vi "Test_URI_Class_SetQuery.vi"(8 "error in (no error)":errorcluster) -> (0 "error out":errorcluster)   [LabVIEW 2013]
uses:
  source/utilities/isHEXDigit.vi
  <vilib>/addons/_JKI Toolkits/Caraya/classes/Assert/Assert Equal Value_Variant.vi
  <vilib>/addons/_JKI Toolkits/Caraya/classes/Assert/Assert True.vi
  source/utilities/Extract URI Components.vi
  <vilib>/Utility/error.llb/Trim Whitespace.vi
  <vilib>/addons/_JKI Toolkits/Caraya/classes/Test/Test.lvclass
  <vilib>/addons/_JKI Toolkits/Caraya/classes/Assert/Assert.lvclass
  source/uri/URI.lvclass
  source/openURI.lvlib
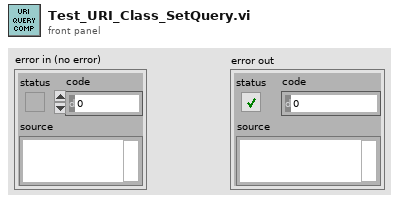
[diagram p1: front panel]
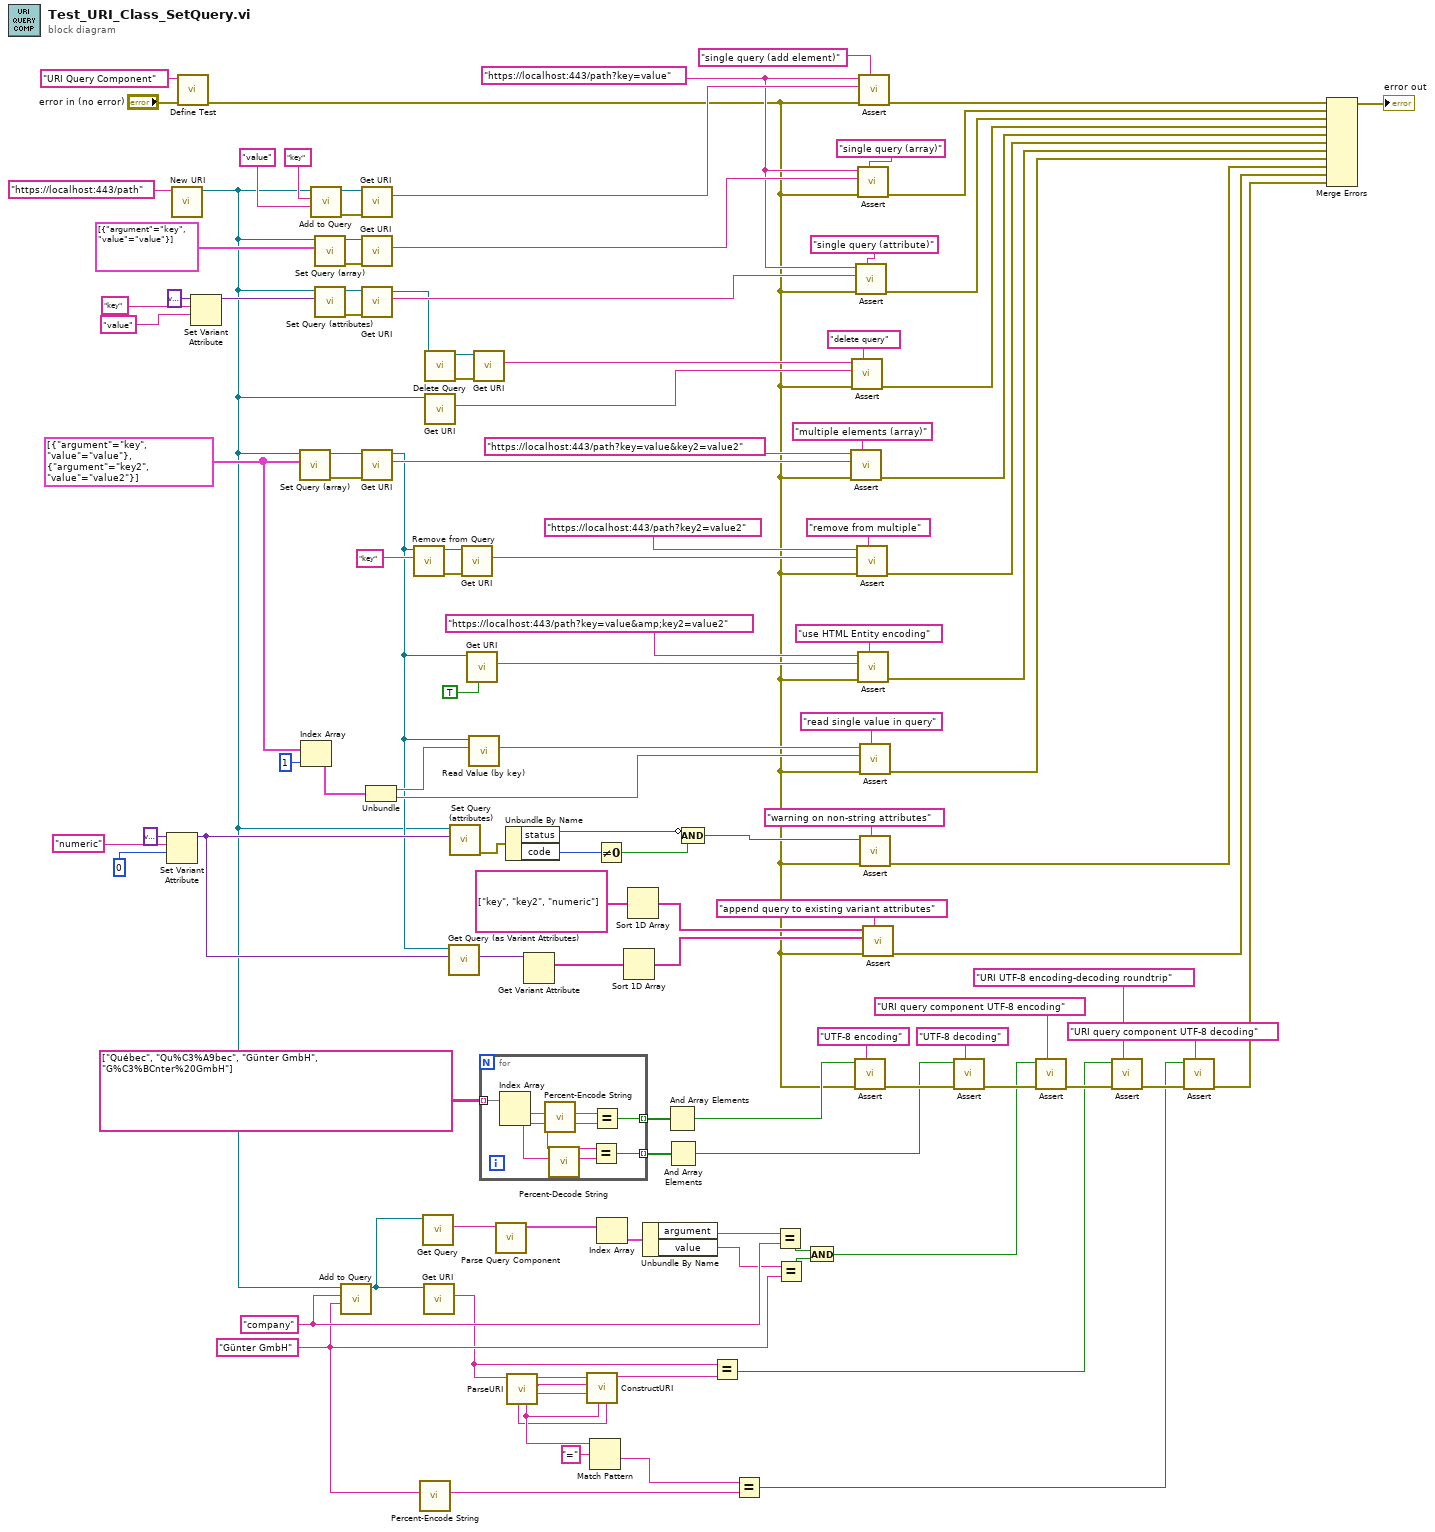
[diagram p0: block diagram]
diagram:
  w22 = "Günter GmbH" ("URI")
  w26 = "company" ("URI")
  w67 = cluster{"argument":string, "value":string}[] [{"argument"="key", "value"="value"}, {"argument"="key2", "value"="value2"}] ("Query")
  w109 = "https://localhost:443/path?key=value" ("URI")
  n1 = Set Variant Attribute(Variant=variant ("variant"), name="numeric" ("URI"), value=0) -> (Variant out=w49:variant)  [unwired: 1 in, 2 out]
  n2 = call "New URI.vi"("URI"="https://localhost:443/path") -> ("URI"=w11:refnum<class "URI.lvclass">)  [unwired: 9 in, 1 out]
  n3 = call <vilib>:"Define Test.vi"("error in (no error)"="error in (no error)", "Label (VI Title)"="URI Query Component") -> ("error out"=w34:errorcluster)  [unwired: 8 in, 1 out]
  n4 = Set Variant Attribute(Variant=variant ("variant"), name="key" ("URI"), value="value") -> (Variant out=w86:variant)  [unwired: 1 in, 2 out]
  n5 = call "Set Query (array).vi"("Query"=w67, "URI in"=w11) -> ("error out"=w79:errorcluster, "URI out"=w80:refnum<class "URI.lvclass">)  [unwired: 8 in]
  n6 = Index Array(array=w67, index=1) -> (element=w65:cluster{"argument":string, "value":string})
  n7 = call "Add to Query.vi"("value"="value" ("URI"), "key"="key" ("URI"), "URI in"=w11) -> ("error out"=w97:errorcluster, "URI out"=w98:refnum<class "URI.lvclass">)  [unwired: 7 in]
  n8 = call "Set Query (array).vi"("Query"=cluster{"argument":string, "value":string}[] [{"argument"="key", "value"="value"}], "URI in"=w11) -> ("error out"=w94:errorcluster, "URI out"=w93:refnum<class "URI.lvclass">)  [unwired: 8 in]
  n9 = call "Set Query (attributes).vi"("Query"=w86, "URI in"=w11) -> ("error out"=w91:errorcluster, "URI out"=w92:refnum<class "URI.lvclass">)  [unwired: 8 in]
  n10 = call "Add to Query.vi"("value"=w22, "key"=w26, "URI in"=w11) -> ("URI out"=w31:refnum<class "URI.lvclass">)  [unwired: 7 in, 1 out]
  n11 = call "Get URI.vi"("error in (no error)"=w97, "URI in"=w98) -> ("URI String"=w113:string)  [unwired: 7 in, 2 out]
  n12 = call "Get URI.vi"("error in (no error)"=w94, "URI in"=w93) -> ("URI String"=w110:string)  [unwired: 7 in, 2 out]
  n13 = call "Get URI.vi"("error in (no error)"=w91, "URI in"=w92) -> ("URI String"=w108:string, "URI"=w85:refnum<class "URI.lvclass">)  [unwired: 7 in, 1 out]
  n14 = call "Get URI.vi"("error in (no error)"=w79, "URI in"=w80) -> ("URI String"=w101:string, "URI"=w48:refnum<class "URI.lvclass">)  [unwired: 7 in, 1 out]
  n15 = Unbundle(w65) -> ("argument"=w64:string, "value"=w61:string)
  n16 = call "Remove from Query.vi"("key"="key" ("argument"), "URI in"=w48) -> ("error out"=w77:errorcluster, "URI out"=w72:refnum<class "URI.lvclass">)  [unwired: 7 in, 1 out]
  n17 = call "Percent-Encode String.vi"("String"=w22) -> ("Pct-Encoded String"=w21:string)  [unwired: 10 in]
  n18 = call "Get Query.vi"("URI in"=w31) -> ("query"=w30:string)  [unwired: 8 in, 2 out]
  n19 = call "Get URI.vi"("URI in"=w31) -> ("URI String"=w12:string)  [unwired: 8 in, 2 out]
  n20 = call "Delete Query.vi"("URI in"=w85) -> ("error out"=w84:errorcluster, "URI out"=w83:refnum<class "URI.lvclass">)  [unwired: 9 in]
  n21 = call "Get URI.vi"("URI in"=w11) -> ("URI String"=w81:string)  [unwired: 8 in, 2 out]
  n22 = call "Get Query (as Variant Attributes).vi"("Container (default: new variant)"=w49, "URI in"=w48) -> ("Container with Query Attributes"=w47:variant)  [unwired: 7 in, 2 out]
  n23 = call "Set Query (attributes).vi"("Query"=w49, "URI in"=w11) -> ("error out"=w56:errorcluster)  [unwired: 8 in, 1 out]
  n24 = call "Get URI.vi"("error in (no error)"=w77, "URI in"=w72) -> ("URI String"=w76:string)  [unwired: 7 in, 2 out]
  n25 = call "Get URI.vi"("HTML Entity (F)"=TRUE, "URI in"=w48) -> ("URI String"=w71:string)  [unwired: 7 in, 2 out]
  n26 = call "Read Value (by key).vi"("key"=w64, "URI in"=w48) -> ("value"=w62:string)  [unwired: 6 in, 3 out]
  n27 = call "Get URI.vi"("error in (no error)"=w84, "URI in"=w83) -> ("URI String"=w82:string)  [unwired: 7 in, 2 out]
  n28 = for {
    tunnel: [w126] -> w39 mode=indexing
    tunnel: string[][] [["Québec", "Qu%C3%A9bec"], ["Günter GmbH", "G%C3%BCnter%20GmbH"]] -> [w124] mode=indexing
    tunnel: [w120] -> w36 mode=indexing
    n29 = Index Array(array=w124) -> (element #1=w121:string, element #2=w123:string)  [unwired: 2 in]
    n30 = call "Percent-Encode String.vi"("String"=w121) -> ("Pct-Encoded String"=w125:string)  [unwired: 10 in]
    n31 = call "Percent-Decode String.vi"("Pct-Encoded String"=w123) -> ("String"=w122:string)  [unwired: 10 in]
    n32 = Equal?(x=w121, y=w122) -> (x = y?=w120:bool)
    n33 = Equal?(x=w125, y=w123) -> (x = y?=w126:bool)
  }
  n34 = call "Parse Query Component.vi"("query"=w30) -> ("Query"=w29:cluster{"argument":string, "value":string}[])  [unwired: 10 in]
  n35 = Unbundle By Name(w56) -> ("status"=w52:bool, "code"=w54:i32)
  n36 = call "ParseURI.vi"("URI"=w12) -> ("path"=w16:string, "authority"=w15:string, "scheme"=w14:string, "query"=w18:string, "fragment"=w17:string)  [unwired: 5 in, 1 out]
  n37 = Get Variant Attribute(Variant=w47) -> (names=w45:string[])  [unwired: 3 in, 3 out]
  n38 = call "ConstructURI.vi"("fragment"=w17, "query"=w18, "path component"=w16, "authority"=w15, "scheme"=w14) -> ("URI"=w13:string)  [unwired: 5 in, 1 out]
  n39 = Match Pattern(string=w18, regular expression="=") -> (after substring=w19:string)  [unwired: 1 in, 3 out]
  n40 = Not Equal To 0?(x=w54) -> (x != 0?=w53:bool)
  n41 = Index Array(array=w29) -> (element=w28:cluster{"argument":string, "value":string})  [unwired: 1 in]
  n42 = Sort 1D Array(array=w45) -> (sorted array=w42:string[])
  n43 = Sort 1D Array(array=string[] ["key", "key2", "numeric"] ("names")) -> (sorted array=w43:string[])
  n44 = Unbundle By Name(w28) -> ("argument"=w27:string, "value"=w25:string)
  n45 = And Array Elements(Boolean array=w39) -> (logical AND=w38:bool)
  n46 = And Array Elements(Boolean array=w36) -> (logical AND=w32:bool)
  n47 = Compound Arithmetic op=AND(invert w52, w53) -> (w51:bool)
  n48 = Equal?(x=w12, y=w13) -> (x = y?=w4:bool)
  n49 = Equal?(x=w19, y=w21) -> (x = y?=w3:bool)
  n50 = Equal?(x=w27, y=w26) -> (x = y?=w23:bool)
  n51 = Equal?(x=w25, y=w22) -> (x = y?=w24:bool)
  n52 = And(x=w23, y=w24) -> (x .and. y?=w9:bool)
  n53 = call-poly <vilib>:"Assert.vi"("Label"="multiple elements (array)" ("URI"), "error in (no error)"=w34, "Y"=w101, "X"="https://localhost:443/path?key=value&key2=value2" ("URI")) -> ("error out"=w102:errorcluster)  [unwired: 6 in, 1 out]
  n54 = call-poly <vilib>:"Assert.vi"("Label"="delete query" ("URI"), "error in (no error)"=w34, "Y"=w81, "X"=w82) -> ("error out"=w104:errorcluster)  [unwired: 6 in, 1 out]
  n55 = call-poly <vilib>:"Assert.vi"("Label"="UTF-8 encoding" ("URI"), "error in (no error)"=w34, "True?"=w38) -> ("error out"=w33:errorcluster)  [unwired: 7 in, 1 out]
  n56 = call-poly <vilib>:"Assert.vi"("Label"="single query (attribute)" ("URI"), "error in (no error)"=w34, "Y"=w108, "X"=w109) -> ("error out"=w106:errorcluster)  [unwired: 6 in, 1 out]
  n57 = call-poly <vilib>:"Assert.vi"("Label"="remove from multiple" ("URI"), "error in (no error)"=w34, "Y"=w76, "X"="https://localhost:443/path?key2=value2" ("URI")) -> ("error out"=w99:errorcluster)  [unwired: 6 in, 1 out]
  n58 = call-poly <vilib>:"Assert.vi"("Label"="single query (array)" ("URI"), "error in (no error)"=w34, "Y"=w110, "X"=w109) -> ("error out"=w107:errorcluster)  [unwired: 6 in, 1 out]
  n59 = call-poly <vilib>:"Assert.vi"("Label"="use HTML Entity encoding" ("URI"), "error in (no error)"=w34, "Y"=w71, "X"="https://localhost:443/path?key=value&amp;key2=value2" ("URI")) -> ("error out"=w68:errorcluster)  [unwired: 6 in, 1 out]
  n60 = call-poly <vilib>:"Assert.vi"("Label"="single query (add element)" ("URI"), "error in (no error)"=w34, "Y"=w113, "X"=w109) -> ("error out"=w114:errorcluster)  [unwired: 6 in, 1 out]
  n61 = call-poly <vilib>:"Assert.vi"("Label"="read single value in query" ("URI"), "error in (no error)"=w34, "Y"=w61, "X"=w62) -> ("error out"=w60:errorcluster)  [unwired: 6 in, 1 out]
  n62 = call-poly <vilib>:"Assert.vi"("Label"="warning on non-string attributes" ("URI"), "error in (no error)"=w34, "True?"=w51) -> ("error out"=w50:errorcluster)  [unwired: 7 in, 1 out]
  n63 = call-poly <vilib>:"Assert.vi"("Label"="append query to existing variant attributes" ("URI"), "error in (no error)"=w34, "Y"=w42, "X"=w43) -> ("error out"=w41:errorcluster)  [unwired: 6 in, 1 out]
  n64 = call-poly <vilib>:"Assert.vi"("Label"="UTF-8 decoding" ("URI"), "error in (no error)"=w33, "True?"=w32) -> ("error out"=w10:errorcluster)  [unwired: 7 in, 1 out]
  n65 = call-poly <vilib>:"Assert.vi"("Label"="URI query component UTF-8 encoding" ("URI"), "error in (no error)"=w10, "True?"=w9) -> ("error out"=w7:errorcluster)  [unwired: 7 in, 1 out]
  n66 = call-poly <vilib>:"Assert.vi"("Label"="URI UTF-8 encoding-decoding roundtrip" ("URI"), "error in (no error)"=w7, "True?"=w4) -> ("error out"=w6:errorcluster)  [unwired: 7 in, 1 out]
  n67 = call-poly <vilib>:"Assert.vi"("Label"="URI query component UTF-8 decoding" ("URI"), "error in (no error)"=w6, "True?"=w3) -> ("error out"=w5:errorcluster)  [unwired: 7 in, 1 out]
  n68 = Merge Errors(w114, w107, w106, w104, w102, w99, w68, w60, w50, w41, w5) -> (→"error out":errorcluster)
